vi "Field Draw Targets.vi"(4 "Lado":enum16{"Esquerdo", "Direito"}(ring) caption="Enum", 6 "Draw Targets?":T2, 7 "RobotRef":refnum<class "Robot.lvclass">[](array[class]), 8 "Picture In":picture, 9 "Offset":cluster{"Width":dbl, "Height":dbl}, 10 "Scale":dbl, 11 "Project":T1=enum."VSS") -> (0 "Picture Out":picture, 1 "Offset Out":cluster{"Width":dbl, "Height":dbl}, 2 "Scale Out":dbl)   [LabVIEW 2022 SP3]
uses:
  DrawTargets.ctl
  Robot_class/Robot.lvclass
  Project.ctl
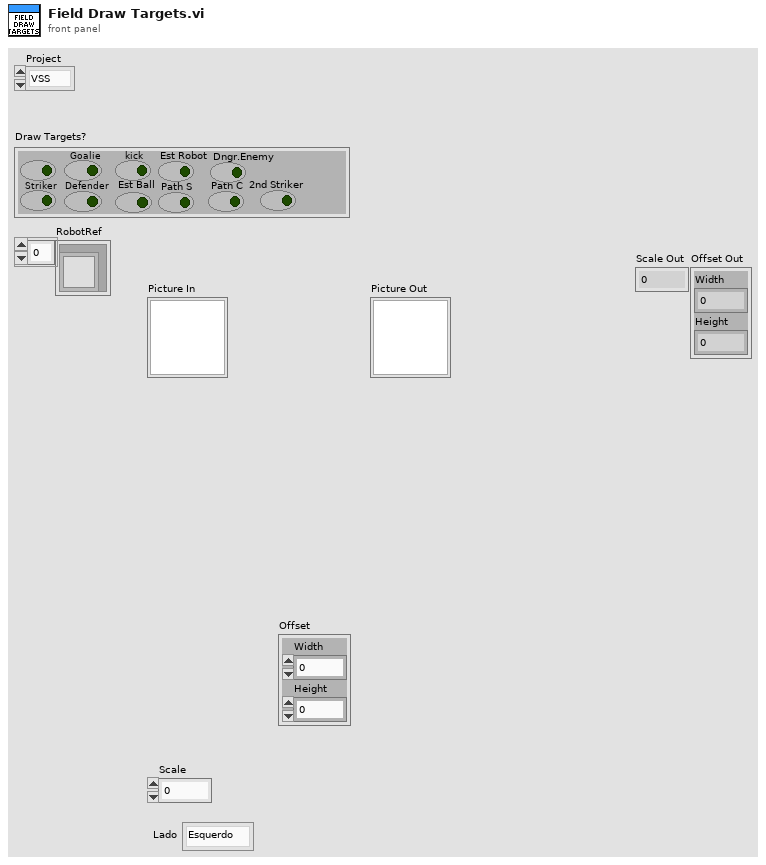
[diagram p1: front panel]
types:
  T1 = typedef "Project.ctl" = enum16{"SSL", "VSS"}
  T2 = typedef "DrawTargets.ctl" = cluster{"Attacker":bool, "Striker":bool, "Goalie":bool, "Defender":bool, "kick":bool, "Est Ball":bool, "Est Robot":bool, "Path S":bool, "Path C":bool, "Dngr.Enemy":bool, "2nd Striker":bool}
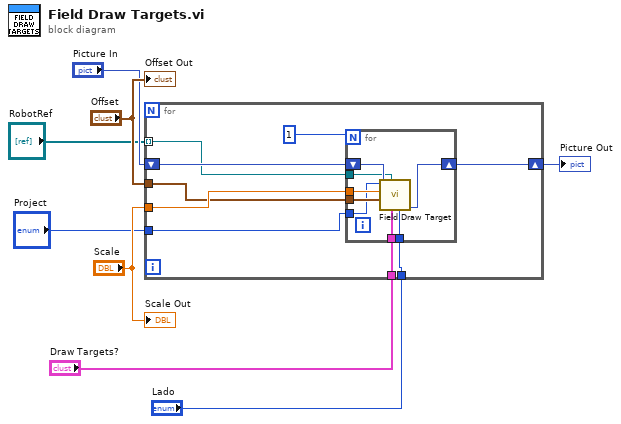
[diagram p0: block diagram]
diagram:
  n1 = for {
    tunnel: "Scale" -> [w17]
    tunnel: "Offset" -> [w15]
    shift-right: [w16] -> w5
    shift-left: "Picture In" -> [w14]
    tunnel: "Draw Targets?" -> [w13]
    tunnel: "Lado" -> [w12]
    tunnel: "RobotRef" -> [w11] mode=indexing
    tunnel: "Project" -> [w9]
    n2 = for {
      N: 1 -> [_]
      tunnel: w17 -> [w25]
      tunnel: w15 -> [w23]
      tunnel: w13 -> [w21]
      tunnel: w12 -> [w20]
      shift-right: [w24] -> w16
      shift-left: w14 -> [w22]
      tunnel: w11 -> [w19]
      tunnel: w9 -> [w18]
      n3 = call "Field Draw Target.vi"("Lado"=w20, "Draw Targets?"=w21, "Robot"=w19, "picture in"=w22, "Offset"=w23, "Scale mm/pixel"=w25, "Project"=w18) -> ("picture out"=w24:picture)  [unwired: 4 in]
    }
  }
  "Picture Out" <- w5
  "Scale Out" <- "Scale"
  "Offset Out" <- "Offset"
